vi "Update Measurements.vi"(0 "OUR Monitor in":refnum<class "OUR_Monitor.lvclass">, 5 "kla":dbl, 7 "So":dbl, 9 "CV":bool, 11 "error in (no error)":errorcluster) -> (4 "OUR Monitor out":refnum<class "OUR_Monitor.lvclass">, 15 "error in (no error) 2":errorcluster)   [LabVIEW 2021, in "MBPOnOff_Controller.lvlib" / "OUR_Monitor.lvclass"]
uses:
  OUR_Monitor.lvclass
  OUR_Monitor.lvclass/OUR_Monitor.ctl
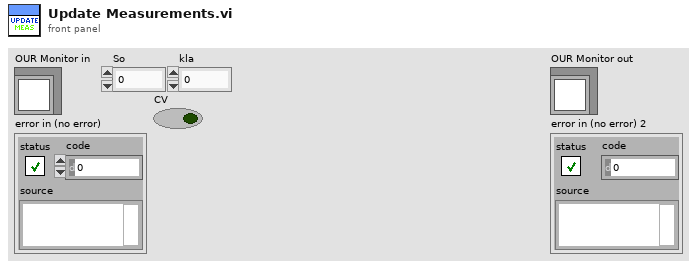
[diagram p1: front panel]
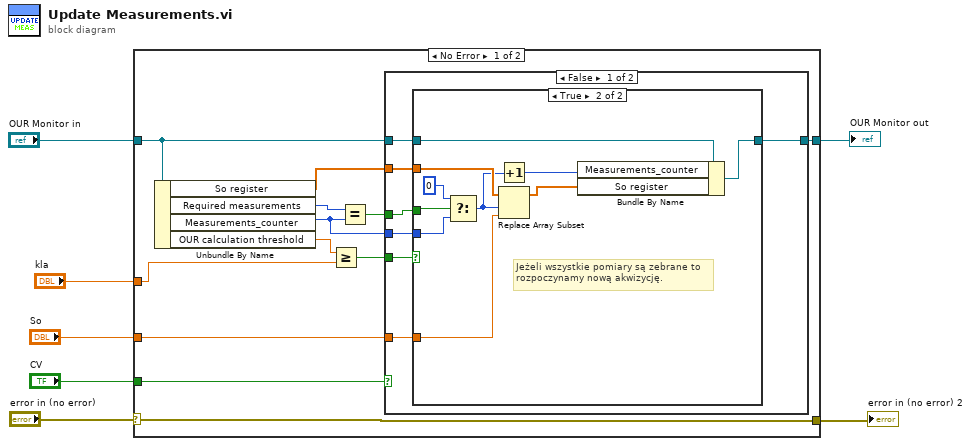
[diagram p0: block diagram]
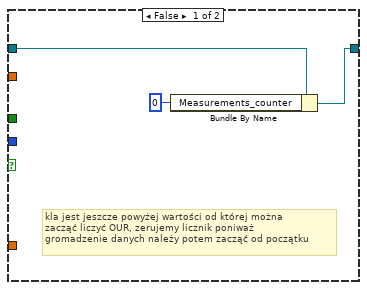
[diagram p2: hidden frame]
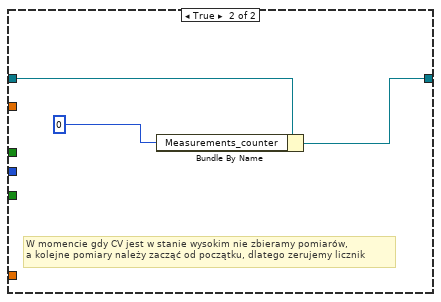
[diagram p3: hidden frame]
diagram:
  n1 = case shown="No Error" "error in (no error)" {
    selector: "error in (no error)" -> [w17 w44]
    tunnel: "OUR Monitor in" -> [w15 w43]
    tunnel: [w17 w44] -> w5
    tunnel: [w14 w43] -> w4
    tunnel: "So" -> [w11 _]
    tunnel: "kla" -> [w18 _]
    tunnel: "CV" -> [w10 _]
    frame No Error {
      n2 = Unbundle By Name(w15) -> ("So register"=w12:dbl[], "Required measurements"=w9:i32, "Measurements_counter"=w8:i32, "OUR calculation threshold"=w19:dbl)
      n3 = Greater Or Equal?(x=w19, y=w18) -> (x >= y?=w16:bool)
      n4 = Equal?(x=w9, y=w8) -> (x = y?=w13:bool)
      n5 = case shown="False" w10 {
        tunnel: w16 -> [w26 _]
        tunnel: w15 -> [w25 w42]
        tunnel: [w24 w41] -> w14
        tunnel: w13 -> [w23 _]
        tunnel: w12 -> [w22 _]
        tunnel: w11 -> [w21 _]
        tunnel: w8 -> [w20 _]
        frame False {
          n6 = case shown="True" w26 {
            tunnel: w25 -> [w29 w39]
            tunnel: [w27 w36] -> w24
            tunnel: w23 -> [_ w33]
            tunnel: w22 -> [_ w38]
            tunnel: w21 -> [_ w37]
            tunnel: w20 -> [_ w30]
            frame False {
              # "kla jest jeszcze powyżej wartości od której można\nzacząć liczyć OUR, zerujemy licznik poniważ\ngromadzenie danych należy potem zacząć od początku"
              n7 = Bundle By Name(cluster=w29, "Measurements_counter"=0) -> (w27:refnum<class "OUR_Monitor.lvclass">)
            }
            frame True {
              # "Jeżeli wszystkie pomiary są zebrane to\nrozpoczynamy nową akwizycję."
              n8 = Select(t=0 ("index"), s=w33, f=w30) -> (s? t:f=w32:i32)
              n9 = Increment(x=w32) -> (x+1=w34:i32)
              n10 = Replace Array Subset(array=w38, new element=w37, index=w32) -> (w35:dbl[])
              n11 = Bundle By Name(cluster=w39, "Measurements_counter"=w34, "So register"=w35) -> (w36:refnum<class "OUR_Monitor.lvclass">)
            }
          }
        }
        frame True {
          # "W momencie gdy CV jest w stanie wysokim nie zbieramy pomiarów, \na kolejne pomiary należy zacząć od początku, dlatego zerujemy licznik"
          n12 = Bundle By Name(cluster=w42, "Measurements_counter"=0) -> (w41:refnum<class "OUR_Monitor.lvclass">)
        }
      }
    }
    frame Error {
    }
  }
  "OUR Monitor out" <- w4
  "error in (no error) 2" <- w5
